vi "Update.vi"(8 "error in (no error)":errorcluster, 11 "NI RIO in":refnum<class "NI RIO.lvclass">) -> (0 "error out":errorcluster, 3 "NI RIO out":refnum<class "NI RIO.lvclass">)   [LabVIEW 2020, in "NI RIO.lvlib" / "NI RIO.lvclass"]
uses:
  NI RIO.lvclass
  NI RIO.lvclass/NI RIO.ctl
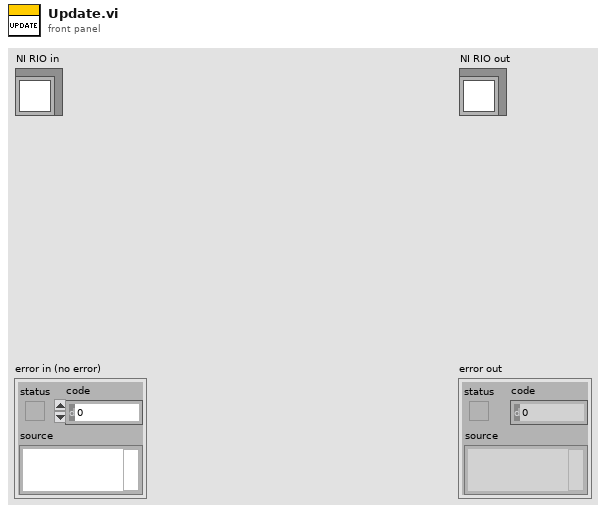
[diagram p1: front panel]
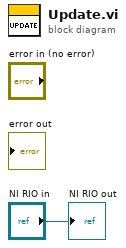
[diagram p0: block diagram]
diagram:
  "NI RIO out" <- "NI RIO in"
